vi "Write Unique Identifier.vi"(8 "error in (no error)":errorcluster, 10 "Unique Identifier":string, 11 "Function Done in":refnum<class "Function Done.lvclass">) -> (0 "error out":errorcluster, 3 "Function Done out":refnum<class "Function Done.lvclass">)   [LabVIEW 2016, in "Controller Actor.lvlib" / "Function Done.lvclass"]
uses:
  <userlib>/Common Components/Controller/Messages/Function Done Message/Function Done.lvclass
  <userlib>/Common Components/Controller/Messages/Function Done Message/Function Done.lvclass/Function Done.ctl
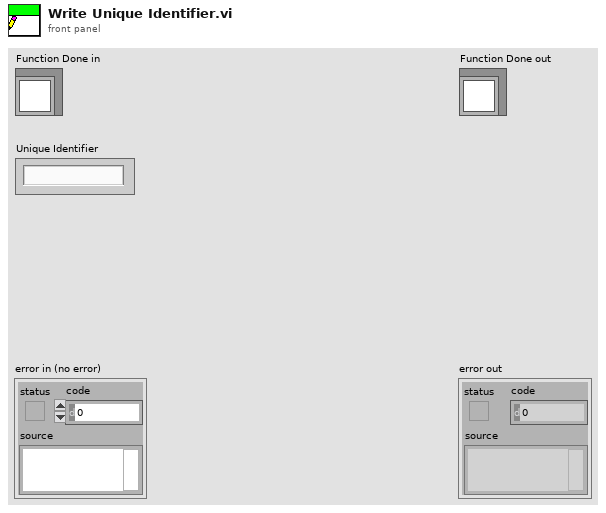
[diagram p1: front panel]
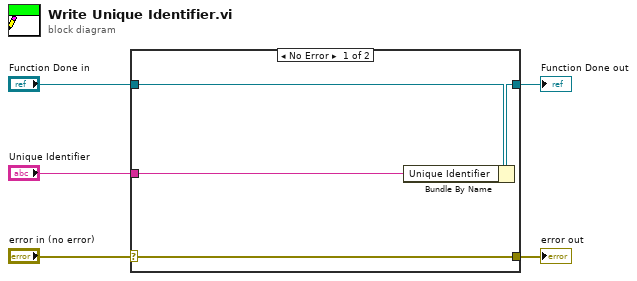
[diagram p0: block diagram]
diagram:
  n1 = case shown="No Error" "error in (no error)" {
    selector: "error in (no error)" -> [w9 w10]
    tunnel: [w9 w10] -> w4
    tunnel: [w7 w11] -> w2
    tunnel: "Function Done in" -> [w8 w11]
    tunnel: "Unique Identifier" -> [w6 _]
    frame No Error {
      n2 = Bundle By Name(cluster=w8, "Unique Identifier"=w6) -> (w7:refnum<class "Function Done.lvclass">)
    }
    frame Error {
    }
  }
  "error out" <- w4
  "Function Done out" <- w2
